vi "HRM-AQN-filter_waveform.vi"(10 "Additional Signal to remove [s]":i32, 11 "data in":waveform(dbl)) -> (3 "data out":waveform(dbl))   [LabVIEW 2020]
uses:
  <vilib>/Analysis/3filter.llb/Filter Passband Type.ctl
  <vilib>/Analysis/3filter.llb/Butterworth Filter (DBL).vi
  <vilib>/Analysis/NI_AALBase.lvlib
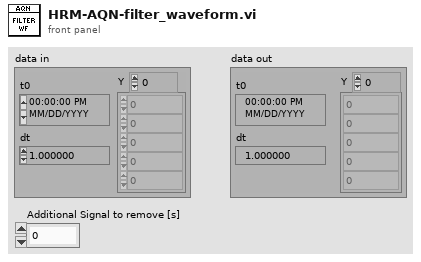
[diagram p1: front panel]
types:
  T1 = typedef "NI_AALBase.lvlib/Filter Passband Type.ctl" = enum32{"Lowpass", "Highpass", "Bandpass", "Bandstop"}
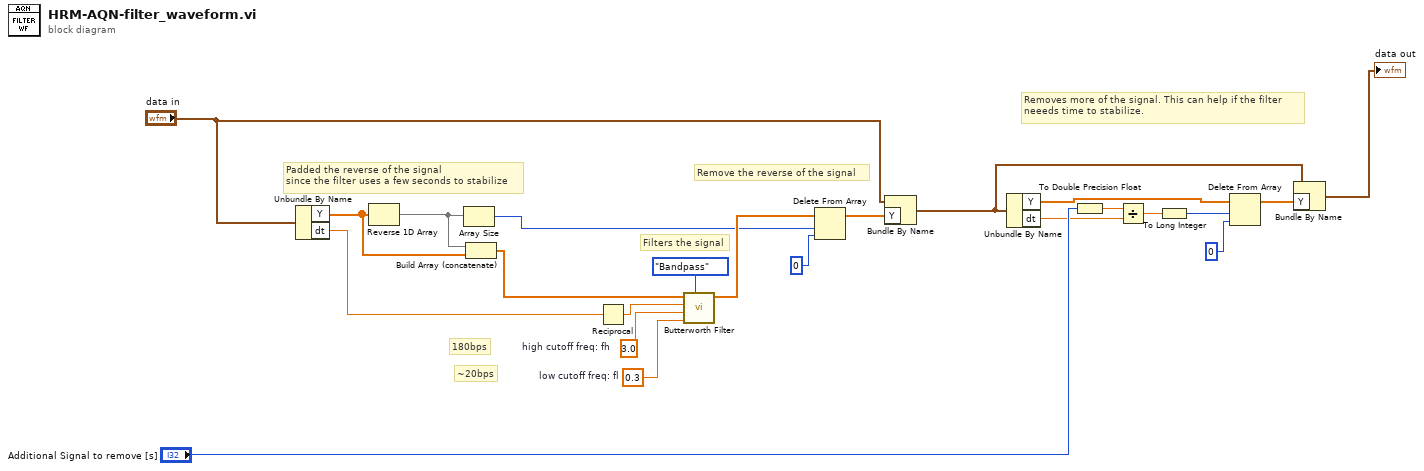
[diagram p0: block diagram]
diagram:
  w22 = 0.3  # low cutoff freq: fl
  w21 = 3.0  # high cutoff freq: fh
  # "Remove the reverse of the signal"
  # "Padded the reverse of the signal\nsince the filter uses a few seconds to stabilize"
  # "Removes more of the signal. This can help if the filter\nneeeds time to stabilize."
  # "Filters the signal"
  # "~20bps"
  # "180bps"
  n1 = Unbundle By Name("data in") -> ("Y"=w7:dbl[], "dt"=w19:dbl)
  n2 = Reverse 1D Array(array=w7) -> (reversed array=w2:dbl[])
  n3 = Array Size(array=w2) -> (size(s)=w1:i32)
  n4 = Build Array (concatenate)(w2, w7) -> (w6:dbl[])
  n5 = Reciprocal(x=w19) -> (1/x=w20:dbl)
  n6 = call-poly <vilib>:"Butterworth Filter.vi"("filter type"=Filter_Passband_Type."Bandpass", "low cutoff freq: fl"=w22, "high cutoff freq: fh"=w21, "sampling freq: fs"=w20, "X"=w6) -> ("Filtered X"=w4:dbl[])  [unwired: 3 in, 1 out]
  n7 = Delete From Array(array=w4, length=w1, index=0) -> (array with subset deleted=w3:dbl[])  [unwired: 1 out]
  n8 = Bundle By Name(cluster="data in", "Y"=w3) -> (w9:waveform(dbl))
  n9 = Unbundle By Name(w9) -> ("Y"=w11:dbl[], "dt"=w13:dbl)
  n10 = To Double Precision Float(number="Additional Signal to remove [s]") -> (double precision float=w16:dbl)
  n11 = Divide(x=w16, y=w13) -> (x/y=w17:dbl)
  n12 = To Long Integer(number=w17) -> (32bit integer=w12:i32)
  n13 = Delete From Array(array=w11, length=w12, index=0) -> (array with subset deleted=w10:dbl[])  [unwired: 1 out]
  n14 = Bundle By Name(cluster=w9, "Y"=w10) -> (→"data out":waveform(dbl))
